vi "Init.vi"(8 "error in (no error)":errorcluster caption="Fehler (Eingang, kein Fehler)", 10 "Main Vi Reference 2":refnum<vi>, 11 "ApplicationInititialisation Eingang":refnum<class "ApplicationInititialisation.lvclass"> caption="DNL_LabVIEW Object in") -> (0 "error out":errorcluster caption="Fehler (Ausgang)", 1 "WhereIGetMyInformation":string, 2 "WhoIAm":string, 3 "ApplicationInititialisation Ausgang":refnum<class "ApplicationInititialisation.lvclass"> caption="DNL_LabVIEW Object out", 4 "Pfad":path)   [LabVIEW 2013, in "ApplicationInititialisation.lvclass"]
uses:
  ApplicationInititialisation.lvclass
  ApplicationInititialisation.lvclass/ApplicationInititialisation.ctl
  <vilib>/Utility/config.llb/Read Key (String).vi
  <vilib>/Utility/config.llb/NI_LVConfig.lvlib
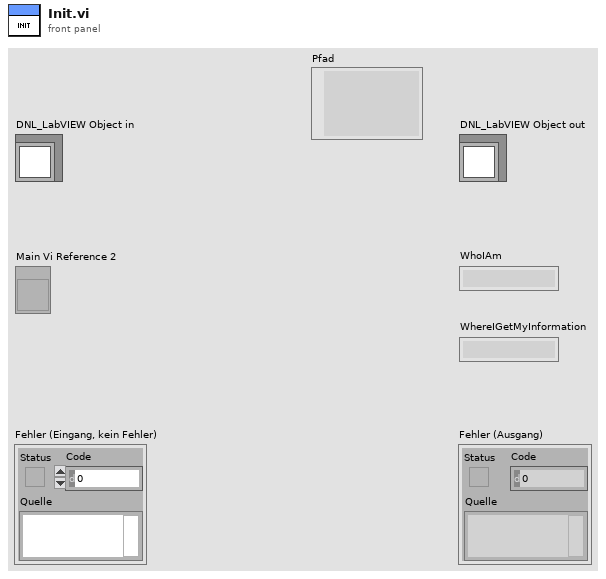
[diagram p1: front panel]
types:
  T1 = typedef "NI_LVConfig.lvlib/Config Data RefNum.ctl" = refnum<k1>
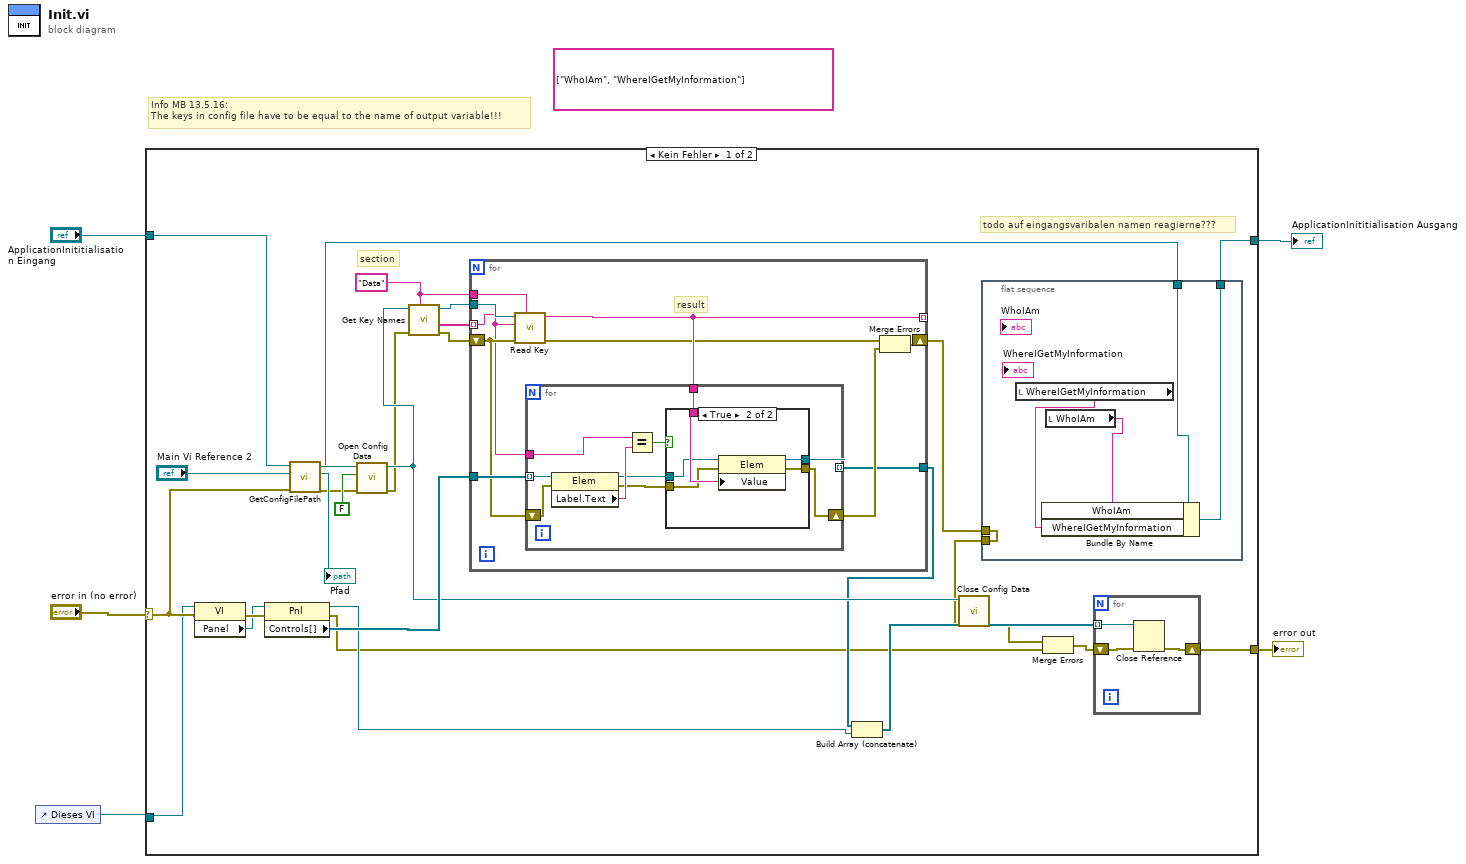
[diagram p0: block diagram]
diagram:
  (unwired) string[] ["WhoIAm", "WhereIGetMyInformation"]
  # "Info MB 13.5.16:\nThe keys in config file have to be equal to the name of output variable!!!"
  n1 = control-ref of="Dieses VI"() -> (w1:refnum<vi>)
  n2 = case shown="Kein Fehler" "error in (no error)" {
    selector: "error in (no error)" -> [w24 w69]
    tunnel: [w6 w69] -> w4
    tunnel: [w26 w68] -> w2
    tunnel: "ApplicationInititialisation Eingang" -> [w31 w68]
    tunnel: w1 -> [w23 _]
    frame No Error {
      w17 = "Data" ("section")
      # "section"
      # "todo auf eingangsvaribalen namen reagierne???"
      n3 = property class="VI"(reference=w23, error in=w24) -> (error out=w22:errorcluster, "Panel"=w21:refnum<vi>)  [unwired: 1 out]
      n4 = property class="Pnl"(reference=w21, error in=w22) -> (reference out=w12:refnum<vi>, error out=w8:errorcluster, "Controls[]"=w20:refnum<vi>[])
      n5 = call-dynamic "GetConfigFilePath.vi"("error in (no error)"=w24, "Main Vi Reference"="Main Vi Reference 2", "ApplicationInititialisation Eingang"=w31) -> ("error out"=w28:errorcluster, "Pfad"=w30:path, "ApplicationInititialisation Ausgang"=w27:refnum<class "ApplicationInititialisation.lvclass">)  [unwired: 6 in]
      "Pfad" <- w30
      n6 = call <vilib>:"Open Config Data.vi"("error in (no error)"=w28, "create file if necessary (T)"=FALSE, "configuration file path"=w30) -> ("error out"=w14:errorcluster, "refnum"=w19:T1)  [unwired: 6 in, 1 out]
      n7 = call <vilib>:"Get Key Names.vi"("section"=w17, "error in (no error)"=w14, "refnum"=w19) -> ("error out"=w15:errorcluster, "key names"=w18:string[], "refnum out"=w16:T1)  [unwired: 5 in, 1 out]
      n8 = for {
        shift-right: [w44] -> w25
        shift-left: w15 -> [w47]
        tunnel: [w49] -> _ mode=indexing
        tunnel: w16 -> [w50]
        tunnel: w20 -> [w48]
        tunnel: w18 -> [w43] mode=indexing
        tunnel: w17 -> [w42]
        tunnel: [w41] -> w13
        # "result"
        n9 = call-poly <vilib>:"Read Key.vi"("section"=w42, "error in (no error)"=w47, "key"=w43, "refnum"=w50) -> ("error out"=w46:errorcluster, "value"=w49:string)  [unwired: 4 in, 2 out]
        n10 = for {
          tunnel: w43 -> [w60]
          tunnel: w49 -> [w58]
          tunnel: w48 -> [w55] mode=indexing
          shift-right: [w52] -> w45
          shift-left: w47 -> [w54]
          tunnel: [w51] -> w41 mode=indexing
          n11 = property class="Elem"(reference=w55, error in=w54) -> (reference out=w56:refnum<vi>, error out=w53:errorcluster, "Label.Text"=w57:string)
          n12 = Equal?(x=w60, y=w57) -> (x = y?=w59:bool)
          n13 = case shown="True" w59 {
            tunnel: w58 -> [_ w67]
            tunnel: w56 -> [w61 w66]
            tunnel: w53 -> [w62 w65]
            tunnel: [w62 w64] -> w52
            tunnel: [w61 w63] -> w51
            frame False {
            }
            frame True {
              n14 = property class="Elem"(reference=w66, error in=w65, "Value"=w67) -> (reference out=w63:refnum<vi>, error out=w64:errorcluster)
            }
          }
        }
        n15 = Merge Errors(w46, w45) -> (w44:errorcluster)
      }
      n16 = Build Array (concatenate)(w13, w12) -> (w11:refnum<vi>[])
      n17 = call <vilib>:"Close Config Data.vi"("error in (no error)"=w10, "refnum"=w19) -> ("error out"=w9:errorcluster)  [unwired: 8 in, 1 out]
      n18 = flat-sequence {
        tunnel: w27 -> [w40]
        tunnel: [w39] -> w26
        tunnel: w25 -> [w36]
        tunnel: [w36] -> w10
        frame #0 {
          n19 = local read "WhereIGetMyInformation"() -> (w37:string)
          n20 = local read "WhoIAm"() -> (w38:string)
          n21 = Bundle By Name(cluster=w40, "WhoIAm"=w38, "WhereIGetMyInformation"=w37) -> (w39:refnum<class "ApplicationInititialisation.lvclass">)
        }
      }
      n22 = Merge Errors(w9, w8) -> (w7:errorcluster)
      n23 = for {
        tunnel: w11 -> [w35] mode=indexing
        shift-right: [w33] -> w6
        shift-left: w7 -> [w34]
        n24 = Close Reference(reference=w35, error in (no error)=w34) -> (error out=w33:errorcluster)
      }
    }
    frame Error {
    }
  }
  "error out" <- w4
  "ApplicationInititialisation Ausgang" <- w2
